vi "Model Number and Folder Setup.vi"(10 "Network Model Location":path, 11 "All Models Excel Sheet":path) -> (3 "Model Data":string[][](array[string]))   [LabVIEW 2012]
doc: "This VI will create a Archive folder and check to see if there \nis a newer version of the \"Model Information\" excel worksheet.\nIf there is a newer version, it will move the older version to the\nArchive folder, copy the new version to the local machine, and open\nthe excel file and save it as a .csv. This will improve performance the next\ntime the program is run.\n\nIf there is no new version, it will open the .csv file (created above)."
panel:
  # "This VI will create a Archive folder and check to see if there \nis a newer version of the \"Model Information\" excel worksheet.\nIf there is a newer version, it will move the older version to the\nArchive folder, copy the new version to the local machine, and open\nthe excel file and save it as a .csv. This will improve performance the next\ntime the program is run.\n\nIf there is no new version, it will open the .csv file (created above)."
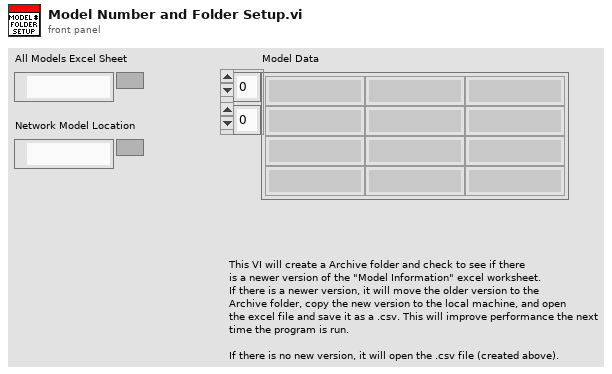
[diagram p1: front panel]
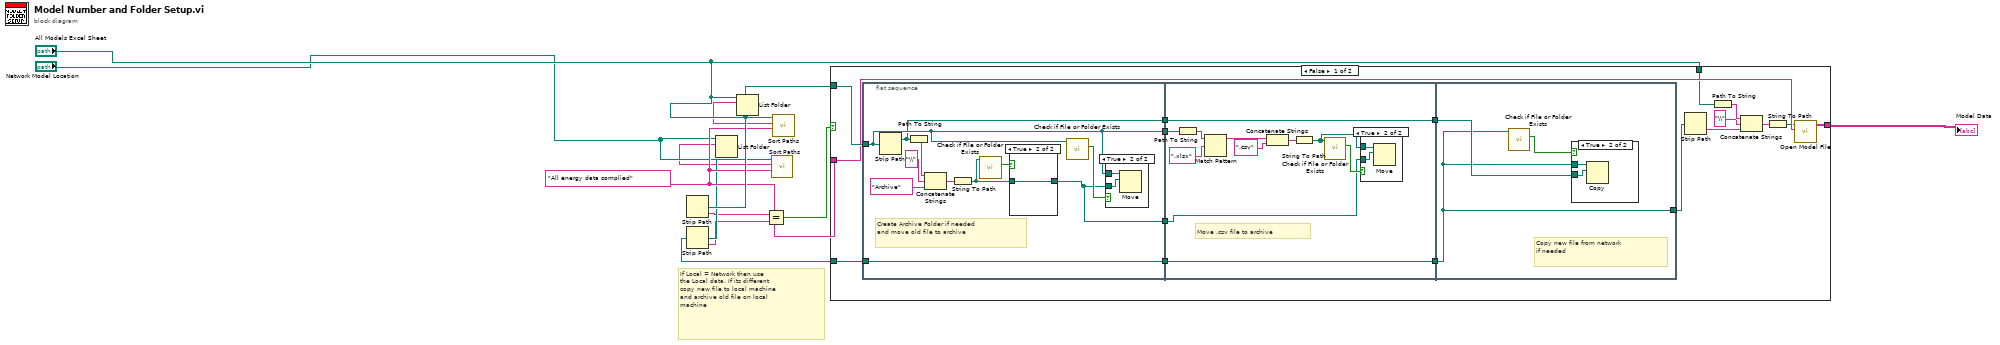
[diagram p0: block diagram]
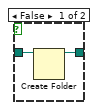
[diagram p3: hidden frame]
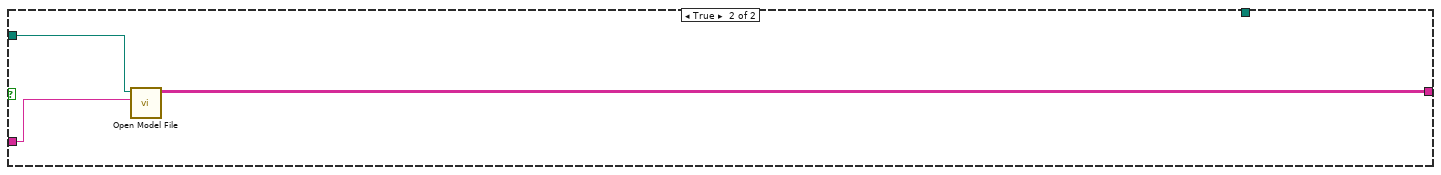
[diagram p6: hidden frame]
diagram:
  w9 = "All energy data complied" ("regular expression")
  # "If Local = Network then use \nthe Local data. If its different \ncopy new file to local machine\nand archive old file on local\nmachine"
  n1 = List Folder(path="Network Model Location") -> (filenames=w1:string[])  [unwired: 3 in, 3 out]
  n2 = List Folder(path="All Models Excel Sheet") -> (filenames=w8:string[])  [unwired: 3 in, 3 out]
  n3 = call "Sort Paths.vi"("Search Expression"=w9, "filenames"=w1, "Folder Path"="Network Model Location") -> ("Latest File on Network Folder"=w7:path)  [unwired: 7 in, 1 out]
  n4 = Strip Path(path=w7) -> (name=w4:string)  [unwired: 1 out]
  n5 = call "Sort Paths.vi"("Search Expression"=w9, "filenames"=w8, "Folder Path"="All Models Excel Sheet") -> ("Latest File on Network Folder"=w10:path)  [unwired: 7 in, 1 out]
  n6 = Strip Path(path=w10) -> (name=w3:string)  [unwired: 1 out]
  n7 = Equal?(x=w3, y=w4) -> (x = y?=w5:bool)
  n8 = case shown="False" w5 {
    tunnel: [w20 w65] -> w6
    tunnel: w10 -> [w28 w64]
    tunnel: w9 -> [w19 w63]
    tunnel: w7 -> [w24 _]
    tunnel: "All Models Excel Sheet" -> [w17 _]
    frame False {
      n9 = flat-sequence {
        tunnel: w28 -> [w32]
        tunnel: [w32] -> w27
        tunnel: [w31] -> w26
        tunnel: [w30] -> w25
        tunnel: w24 -> [w30]
        tunnel: [w29] -> w22
        tunnel: w27 -> [w49]
        tunnel: w26 -> [w48]
        tunnel: w25 -> [w47]
        tunnel: [w47] -> w23
        tunnel: w22 -> [w46]
        tunnel: [w46] -> w21
        tunnel: w23 -> [w58]
        tunnel: w21 -> [w60]
        tunnel: [w58] -> w18
        frame #0 {
          # "Create Archive Folder if needed\nand move old file to archive"
          n10 = Strip Path(path=w32) -> (stripped path=w29:path)  [unwired: 1 out]
          n11 = Path To String(path=w29) -> (string=w34:string)
          n12 = Concatenate Strings(w34, "\\" ("string"), "Archive" ("Search Expression")) -> (w37:string)
          n13 = String To Path(string=w37) -> (path=w39:path)
          n14 = call <vilib>:"Check if File or Folder Exists.vi"("path"=w39) -> ("file or folder exists?"=w38:bool)  [unwired: 8 in, 2 out]
          n15 = case shown="True" w38 {
            tunnel: w39 -> [w43 w44]
            tunnel: [w42 w44] -> w31
            frame False {
              n16 = Create Folder(path (use dialog)=w43) -> (created path=w42:path)  [unwired: 2 in, 2 out]
            }
            frame True {
            }
          }
          n17 = call <vilib>:"Check if File or Folder Exists.vi"("path"=w32) -> ("file or folder exists?"=w33:bool)  [unwired: 8 in, 2 out]
          n18 = case shown="True" w33 {
            tunnel: w31 -> [_ w41]
            tunnel: w32 -> [_ w40]
            frame False {
            }
            frame True {
              n19 = Move(source path=w40, 10:w41) -> ()  [unwired: 3 in, 3 out]
            }
          }
        }
        frame #1 {
          # "Move .csv file to archive"
          n20 = Path To String(path=w49) -> (string=w51:string)
          n21 = Match Pattern(string=w51, regular expression=".xlsx") -> (before substring=w53:string)  [unwired: 1 in, 3 out]
          n22 = Concatenate Strings(w53, ".csv" ("replace string (\"\")")) -> (w55:string)
          n23 = String To Path(string=w55) -> (path=w45:path)
          n24 = call <vilib>:"Check if File or Folder Exists.vi"("path"=w45) -> ("file or folder exists?"=w50:bool)  [unwired: 8 in, 2 out]
          n25 = case shown="True" w50 {
            tunnel: w48 -> [_ w57]
            tunnel: w45 -> [_ w56]
            frame False {
            }
            frame True {
              n26 = Move(source path=w56, 10:w57) -> ()  [unwired: 3 in, 3 out]
            }
          }
        }
        frame #2 {
          # "Copy new file from network\nif needed"
          n27 = call <vilib>:"Check if File or Folder Exists.vi"("path"=w58) -> ("file or folder exists?"=w59:bool)  [unwired: 8 in, 2 out]
          n28 = case shown="True" w59 {
            tunnel: w60 -> [_ w62]
            tunnel: w58 -> [_ w61]
            frame False {
            }
            frame True {
              n29 = Copy(10:w62, 11:w61) -> ()  [unwired: 3 in, 3 out]
            }
          }
        }
      }
      n30 = Strip Path(path=w18) -> (name=w14:string)  [unwired: 1 out]
      n31 = Path To String(path=w17) -> (string=w16:string)
      n32 = Concatenate Strings(w16, "\\" ("string"), w14) -> (w13:string)
      n33 = String To Path(string=w13) -> (path=w12:path)
      n34 = call "Open Model File.vi"("regular expression"=w19, "All Models Excel Sheet"=w12) -> ("all rows"=w20:string[][])  [unwired: 9 in]
    }
    frame True {
      n35 = call "Open Model File.vi"("regular expression"=w63, "All Models Excel Sheet"=w64) -> ("all rows"=w65:string[][])  [unwired: 9 in]
    }
  }
  "Model Data" <- w6
